vi "Write.vi"(8 "error in":errorcluster, 9 "Producer Ch":T2, 10 "Producer Control":T1, 11 "Chiller Cluster.lvclass":refnum<class "Climate Chamber Cluster.lvclass">) -> (0 "error out":errorcluster, 3 "output cluster":refnum<class "Climate Chamber Cluster.lvclass">)   [LabVIEW 2023, in "Climate Chamber Cluster.lvclass"]
uses:
  Climate Chamber Cluster.lvclass
  6bfc6677-cd67-4f2d-afef-839dec9218ce.vi
  74f11eb1-9425-41af-a169-6608e4aa6674.vi
  Producer Ch Array.ctl
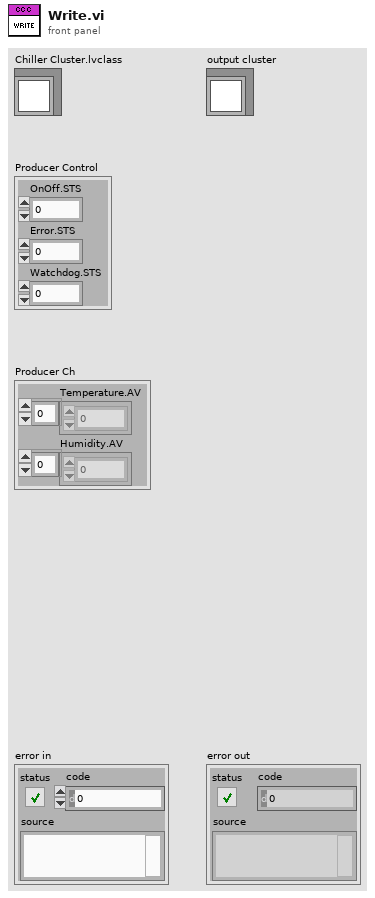
[diagram p1: front panel]
types:
  T1 = cluster{"OnOff.STS":i32, "Error.STS":i32, "Watchdog.STS":i32}
  T2 = typedef "Climate Chamber Cluster.lvclass/Producer Ch Array.ctl" = cluster{"Temperature.AV":dbl[], "Humidity.AV":dbl[]}
  T3 = cluster{"Temperature.ch01.AV":dbl, "Humidity.ch01.AV":dbl}
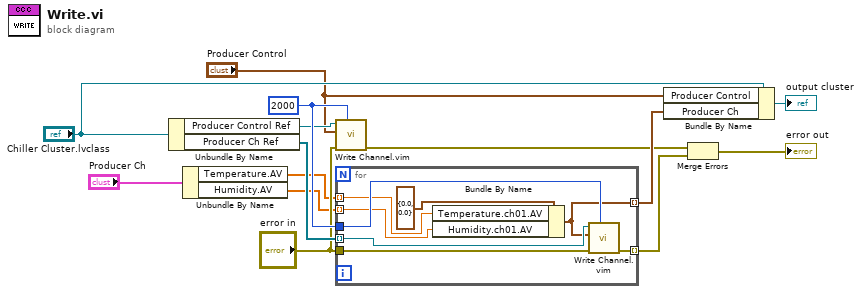
[diagram p0: block diagram]
diagram:
  w11 = 2000 ("Timeout (ms)")
  n1 = Unbundle By Name("Chiller Cluster.lvclass") -> ("Producer Control Ref"=w10:refnum<k21>, "Producer Ch Ref"=w12:refnum<k21>[])
  n2 = Unbundle By Name("Producer Ch") -> ("Temperature.AV"=w1:dbl[], "Humidity.AV"=w2:dbl[])
  n3 = call "Write Channel.vim"("Timeout (ms)"=w11, "error in"="error in", "Data in"="Producer Control", "ADAS HIL Channel in"=w10) -> ("error out"=w7:errorcluster)  [unwired: 5 in, 2 out]
  n4 = for {
    tunnel: [w18] -> w9 mode=indexing
    tunnel: "error in" -> [w22]
    tunnel: [w21] -> w6 mode=indexing
    tunnel: w12 -> [w20] mode=indexing
    tunnel: w11 -> [w19]
    tunnel: w2 -> [w16] mode=indexing
    tunnel: w1 -> [w15] mode=indexing
    n5 = Bundle By Name(cluster=T3 {"Temperature.ch01.AV"=0.0, "Humidity.ch01.AV"=0.0} ("Producer Ch 01"), "Temperature.ch01.AV"=w15, "Humidity.ch01.AV"=w16) -> (w18:T3)
    n6 = call "Write Channel.vim"("Timeout (ms)"=w19, "error in"=w22, "Data in"=w18, "ADAS HIL Channel in"=w20) -> ("error out"=w21:errorcluster)  [unwired: 5 in, 2 out]
  }
  n7 = Bundle By Name(cluster="Chiller Cluster.lvclass", "Producer Control"="Producer Control", "Producer Ch"=w9) -> (→"output cluster":refnum<class "Climate Chamber Cluster.lvclass">)
  n8 = Merge Errors(w7, w6) -> (→"error out":errorcluster)
